vi "Enqueue Acknowledge Message.vi"(7 "Ack Timeout":i32=-1, 8 "error in":errorcluster, 11 "Message Data":T1) -> (0 "error out":errorcluster, 2 "Timed Out":bool, 3 "Response Data":string)   [LabVIEW 2015, in "Generic Module Library.lvlib" / "Template G_Module.lvlib"]
uses:
  Template G_Module.lvlib
  Queue Support/Queue Reference Actions.ctl
  Private Controls/Module Message Cluster Components/Acknowledge Data Cluster.ctl
  Private Controls/Module Message Cluster.ctl
  Private Controls/Module Message Cluster Components/Message Data Cluster.ctl
  Private Controls/Module Message Cluster Components/Ack Payload.ctl
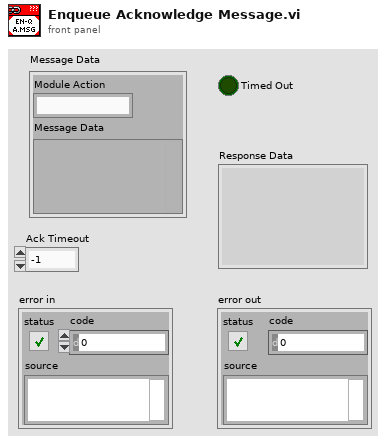
[diagram p1: front panel]
types:
  T1 = typedef "Generic Module Library.lvlib/Template G_Module.lvlib/Message Data Cluster.ctl" = cluster{"Module Action":string, "Message Data":variant}
  T2 = typedef "Generic Module Library.lvlib/Template G_Module.lvlib/Module Message Cluster.ctl" = cluster{"Message Data":T1, "Acknowledge Data":T3}
  T3 = typedef "Generic Module Library.lvlib/Template G_Module.lvlib/Acknowledge Data Cluster.ctl" = cluster{"Ack Requested":bool, "Ack Notifier Ref":refnum<notifier>, "Response Payload":T4}
  T4 = typedef "Generic Module Library.lvlib/Template G_Module.lvlib/Ack Payload.ctl" = cluster{"Response Data":string, "error out":errorcluster}
  T5 = typedef "Generic Module Library.lvlib/Template G_Module.lvlib/Queue Reference Actions.ctl" = enum16{"Release", "Set", "Get"}
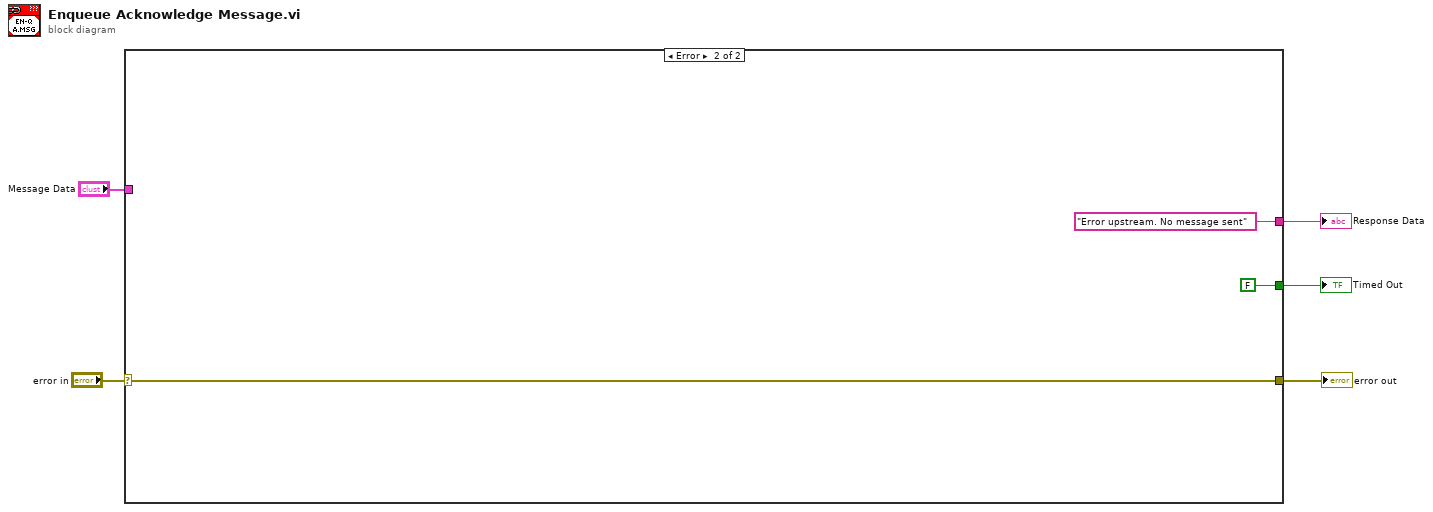
[diagram p0: block diagram]
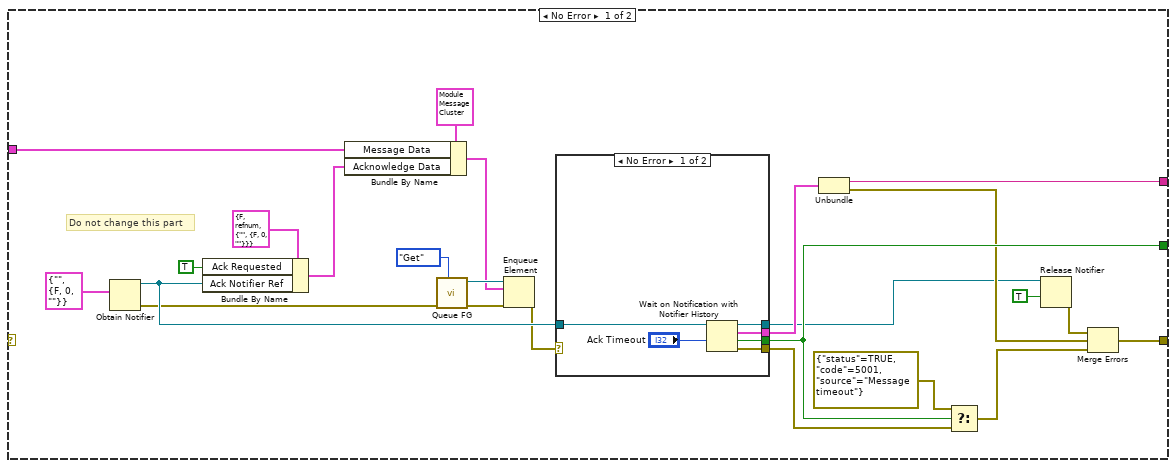
[diagram p2: hidden frame]
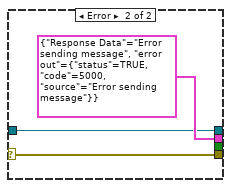
[diagram p3: hidden frame]
diagram:
  n1 = case shown="Error" "error in" {
    selector: "error in" -> [_ w41]
    tunnel: "Message Data" -> [w20 _]
    tunnel: [w19 FALSE ("timed out?")] -> w4
    tunnel: [w15 "Error upstream. No message sent" ("Response Data")] -> w3
    tunnel: [w13 w41] -> w2
    frame No Error {
      # "Do not change this part"
      n2 = Obtain Notifier(notification data type=T4 {"Response Data"="", "error out"={"status"=FALSE, "code"=0, "source"=""}} ("Payload")) -> (notifier out=w17:refnum<notifier>, error out=w9:errorcluster)  [unwired: 3 in, 1 out]
      n3 = Bundle By Name(cluster=T3 {"Ack Requested"=FALSE, "Ack Notifier Ref"=refnum, "Response Payload"={"Response Data"="", "error out"={"status"=FALSE, "code"=0, "source"=""}}} ("Acknowledge Data"), "Ack Requested"=TRUE, "Ack Notifier Ref"=w17) -> (w22:T3)
      n4 = Bundle By Name(cluster=T2 {"Message Data"={"Module Action"="", "Message Data"=variant}, "Acknowledge Data"={"Ack Requested"=FALSE, "Ack Notifier Ref"=refnum, "Response Payload"={"Response Data"="", "error out"={"status"=FALSE, "code"=0, "source"=""}}}} ("element"), "Message Data"=w20, "Acknowledge Data"=w22) -> (w25:T2)
      n5 = call "Queue FG.vi"("Queue Reference Actions"=Queue_Reference_Actions."Get", "error in"=w9) -> ("error out"=w29:errorcluster, "Queue out"=w28:refnum<queue>)  [unwired: 8 in]
      n6 = Enqueue Element(queue=w28, element=w25, error in (no error)=w29) -> (error out=w11:errorcluster)  [unwired: 1 in, 2 out]
      n7 = case shown="No Error" w11 {
        selector: w11 -> [_ w38]
        tunnel: [w34 w36] -> w10
        tunnel: [w33 _] -> w19
        tunnel: w17 -> [w32 w36]
        tunnel: [w31 T4 {"Response Data"="Error sending message", "error out"={"status"=TRUE, "code"=5000, "source"="Error sending message"}} ("Payload")] -> w16
        tunnel: [w30 w38] -> w8
        frame No Error {
          n8 = Wait on Notification with Notifier History(0:w32, 2:"Ack Timeout") -> (8:w34:refnum<notifier>, 9:w31:T4, 10:w33:bool, 11:w30:errorcluster)  [unwired: 2 in]
        }
        frame Error {
        }
      }
      n9 = Unbundle(w16) -> ("Response Data"=w15:string, "error out"=w12:errorcluster)
      n10 = Select(t=errorcluster {"status"=TRUE, "code"=5001, "source"="Message timeout"} ("error in (no error)"), s=w19, f=w8) -> (s? t:f=w7:errorcluster)
      n11 = Release Notifier(notifier=w10, force destroy? (F)=TRUE) -> (error out=w14:errorcluster)  [unwired: 1 in, 2 out]
      n12 = Merge Errors(w14, w12, w7) -> (w13:errorcluster)
    }
    frame Error {
    }
  }
  "error out" <- w2
  "Timed Out" <- w4
  "Response Data" <- w3
